vi "Scan Engine EtherCAT Slave.vi"(8 "error in (no error)":errorcluster, 11 "Node Ptr":T1 format="%.0x") -> (0 "error out":errorcluster)   [LabVIEW 2016, in "Scan Engine Custom Device.lvlib"]
uses:
  Scan Engine Custom Device.lvlib
  <vilib>/NI Veristand/Custom Device API/Custom Device Item Ref.ctl
  <vilib>/NI Veristand/Custom Device API/Custom Device API.lvlib
panel:
  in  "Prepend":bool caption="Prepend slave position to name"
  in  "SHDocVw.IWebBrowser2":refnum<k7>(container)
  in  "Slave Position":u16
  in  "Header":cluster{"Section Name":string}={"Section Name"="NI-9144 Chassis"}
  in  "Name":string
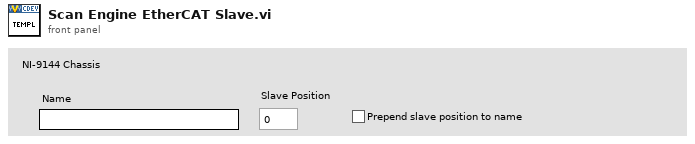
[diagram p1: front panel]
types:
  T1 = typedef "Custom Device API.lvlib/Custom Device Item Ref.ctl" = u64
  T2 = typedef "Custom Device API.lvlib/Custom Device Commands.ctl" = enum16{"Default", "Item renamed", "Shutdown", "Dynamic button pressed"}
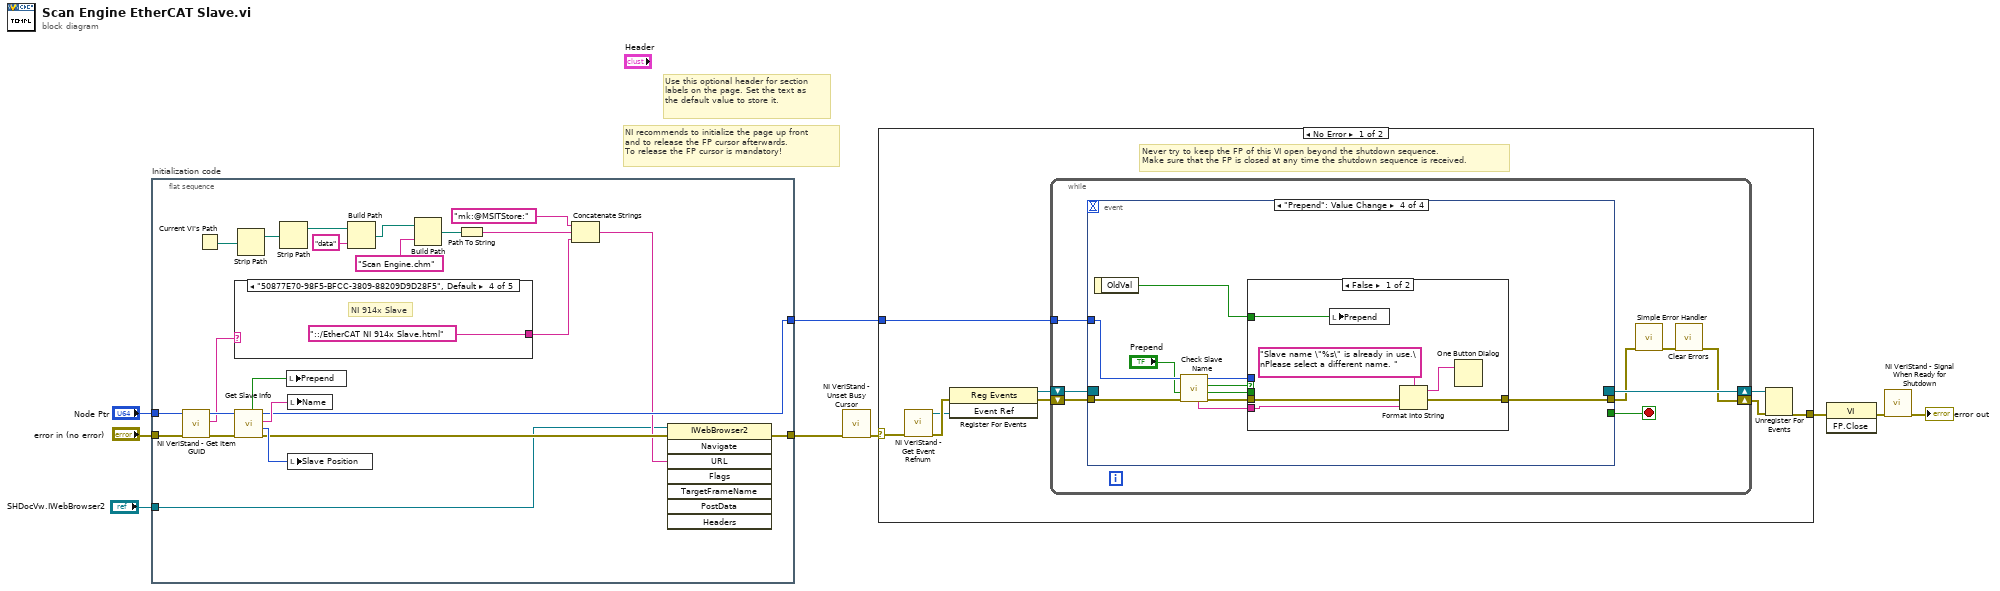
[diagram p0: block diagram]
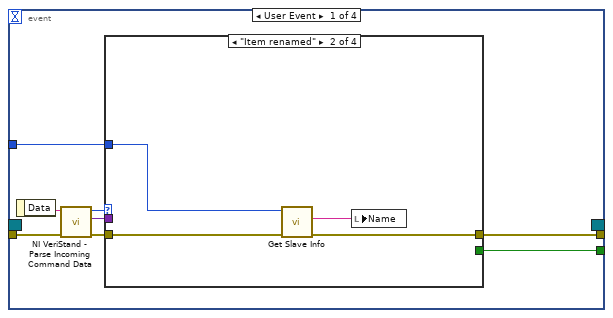
[diagram p2: hidden frame]
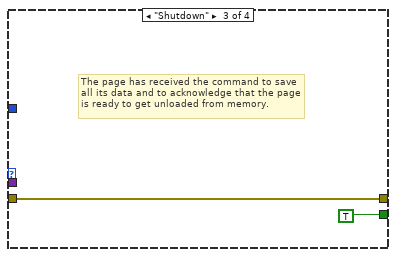
[diagram p4: hidden frame]
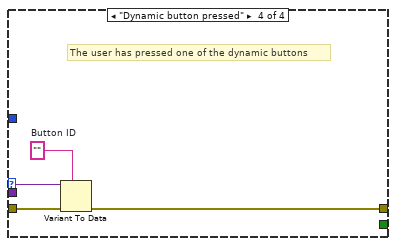
[diagram p5: hidden frame]
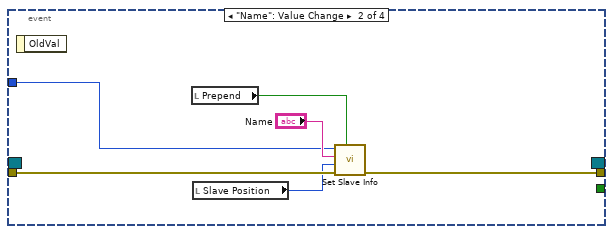
[diagram p6: hidden frame]
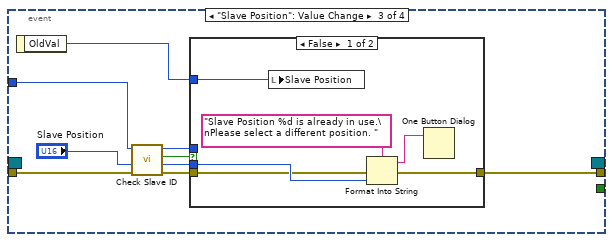
[diagram p7: hidden frame]
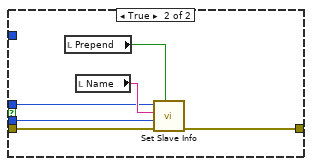
[diagram p8: hidden frame]
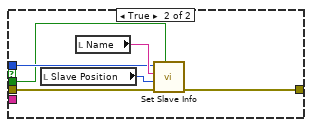
[diagram p9: hidden frame]
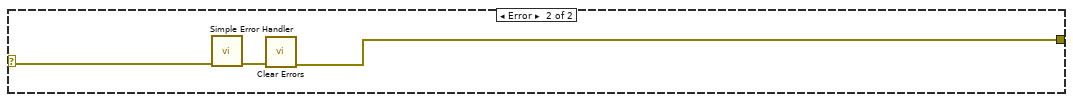
[diagram p10: hidden frame]
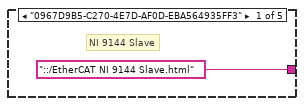
[diagram p11: hidden frame]
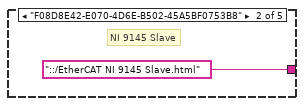
[diagram p12: hidden frame]
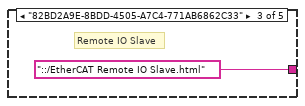
[diagram p13: hidden frame]
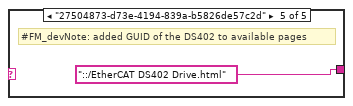
[diagram p14: hidden frame]
diagram:
  # "Use this optional header for section labels on the page. Set the text as the default value to store it."
  # "NI recommends to initialize the page up front\nand to release the FP cursor afterwards.\nTo release the FP cursor is mandatory!"
  n1 = flat-sequence "Initialization code" {
    tunnel: "error in (no error)" -> [w29]
    tunnel: "Node Ptr" -> [w13]
    tunnel: [w18] -> w5
    tunnel: [w30] -> w2
    tunnel: "SHDocVw.IWebBrowser2" -> [w16]
    frame #0 {
      n2 = call <vilib>:"NI VeriStand - Get Item GUID.vi"("error in (no error)"=w29, "Item Ref in"=w13) -> ("error out"=w14:errorcluster, "GUID"=w11:string, "Item Ref out"=w12:T1)  [unwired: 7 in]
      n3 = Current VI's Path() -> (path=w20:path)
      n4 = case shown="\"50877E70-98F5-BFCC-3809-88209D9D28F5\", Default" w11 {
        tunnel: ["::/EtherCAT NI 9144 Slave.html" ("name or relative path") "::/EtherCAT NI 9145 Slave.html" ("name or relative path") "::/EtherCAT Remote IO Slave.html" ("name or relative path") "::/EtherCAT NI 914x Slave.html" ("name or relative path") "::/EtherCAT DS402 Drive.html" ("name or relative path")] -> w10
        frame "0967D9B5-C270-4E7D-AF0D-EBA564935FF3" {
          # "NI 9144 Slave"
        }
        frame "F08D8E42-E070-4D6E-B502-45A5BF0753B8" {
          # "NI 9145 Slave"
        }
        frame "82BD2A9E-8BDD-4505-A7C4-771AB6862C33" {
          # "Remote IO Slave"
        }
        frame "50877E70-98F5-BFCC-3809-88209D9D28F5", Default {
          # "NI 914x Slave"
        }
        frame "27504873-d73e-4194-839a-b5826de57c2d" {
          # "#FM_devNote: added GUID of the DS402 to available pages"
        }
      }
      n5 = call "Get Slave Info.vi"("error in (no error)"=w14, "Item Ref in"=w12) -> ("error out"=w19:errorcluster, "Slave #"=w31:u16, "Slave Name"=w32:string, "Item Ref out"=w30:T1, "Prepend"=w15:bool)  [unwired: 5 in]
      n6 = Strip Path(path=w20) -> (stripped path=w21:path)  [unwired: 1 out]
      n7 = Strip Path(path=w21) -> (stripped path=w26:path)  [unwired: 1 out]
      n8 = local write "Prepend"(w15) -> ()
      n9 = local write "Name"(w32) -> ()
      n10 = local write "Slave Position"(w31) -> ()
      n11 = Build Path(base path=w26, name or relative path="data") -> (appended path=w27:path)
      n12 = Build Path(base path=w27, name or relative path="Scan Engine.chm") -> (appended path=w24:path)
      n13 = Path To String(path=w24) -> (string=w23:string)
      n14 = Concatenate Strings("mk:@MSITStore:" ("string"), w23, w10) -> (w17:string)
      n15 = invoke class="IWebBrowser2" method="Navigate"(reference=w16, error in=w19, "URL"=w17) -> (error out=w18:errorcluster)  [unwired: 5 in, 7 out]
    }
  }
  n16 = call <vilib>:"NI VeriStand - Unset Busy Cursor.vi"("error in (no error)"=w5) -> ("error out"=w4:errorcluster)  [unwired: 10 out]
  n17 = case shown="No Error" w4 {
    selector: w4 -> [w38 w125]
    tunnel: [w43 w123] -> w9
    tunnel: w2 -> [w39 _]
    frame No Error {
      # "Never try to keep the FP of this VI open beyond the shutdown sequence.\nMake sure that the FP is closed at any time the shutdown sequence is received."
      n18 = call <vilib>:"NI VeriStand - Get Event Refnum.vi"("error in (no error)"=w38) -> ("error out"=w46:errorcluster, "Event Ref"=w42:refnum<user-event>)  [unwired: 9 out]
      n19 = register-events(error in=w46, w42) -> (reference out=w40:refnum<event-registration>, error out=w41:errorcluster)  [unwired: 1 in]
      n20 = while {
        tunnel: w39 -> [w50]
        shift-right: [w47] -> w44
        shift-left: w41 -> [w53]
        shift-right: [w54] -> w45
        shift-left: w40 -> [w52]
        stop <- w51 stop-if-true
        n21 = event shown="[3] \"Prepend\": Value Change" {
          selector: w52 -> [_ _ _ _]
          dyn-events: [_ _ _ _] -> w54
          timeout: _ -> [_ _ _ _]
          tunnel: w53 -> [w62 w77 w82 w108]
          tunnel: [w58 _ _ _] -> w51
          tunnel: [w57 w78 w80 w109] -> w49
          tunnel: w50 -> [w56 w76 w84 w107]
          event User Event {
            n22 = event-data() -> ("Data"=w61:string)  [unwired: 1 out]
            n23 = call <vilib>:"NI VeriStand - Parse Incoming Command Data.vi"("error in (no error)"=w62, "Incoming data"=w61) -> ("error out"=w60:errorcluster, "Outgoing data"=w55:variant, "Action"=w59:T2)  [unwired: 7 out]
            n24 = case shown="\"Item renamed\"" w59 {
              tunnel: w60 -> [w63 w67 w68 w73]
              tunnel: [_ _ TRUE _] -> w58
              tunnel: [w63 w66 w68 w70] -> w57
              tunnel: w56 -> [_ w64 _ _]
              tunnel: w55 -> [_ _ _ w72]
              frame "Default", Default {
              }
              frame "Item renamed" {
                n25 = call "Get Slave Info.vi"("error in (no error)"=w67, "Item Ref in"=w64) -> ("error out"=w66:errorcluster, "Slave Name"=w65:string)  [unwired: 5 in, 3 out]
                n26 = local write "Name"(w65) -> ()
              }
              frame "Shutdown" {
                # "The page has received the command to save all its data and to acknowledge that the page is ready to get unloaded from memory."
              }
              frame "Dynamic button pressed" {
                w71 = ""  # Button ID
                # "The user has pressed one of the dynamic buttons"
                n27 = Variant To Data(error in=w73, type=w71, Variant=w72) -> (error out=w70:errorcluster)  [unwired: 1 out]
              }
            }
          }
          event "Name": Value Change {
            n28 = event-data() -> ()  [unwired: 2 out]
            n29 = local read "Prepend"() -> (w74:bool)
            n30 = local read "Slave Position"() -> (w75:u16)
            n31 = call "Set Slave Info.vi"("Prepend"=w74, "error in (no error)"=w77, "Slave #"=w75, "Slave Name"="Name", "Item Ref in"=w76) -> ("error out"=w78:errorcluster)  [unwired: 5 in, 1 out]
          }
          event "Slave Position": Value Change {
            n32 = event-data() -> ("OldVal"=w81:u16)  [unwired: 1 out]
            n33 = call "Check Slave ID.vi"("error in (no error)"=w82, "Slave ID in"="Slave Position", "Item Ref in"=w84) -> ("error out"=w88:errorcluster, "Slave ID out"=w86:u16, "Available?"=w87:bool, "Item Ref out"=w85:T1)  [unwired: 5 in]
            n34 = case shown="False" w87 {
              tunnel: [w90 w100] -> w80
              tunnel: w88 -> [w91 w99]
              tunnel: w85 -> [_ w96]
              tunnel: w86 -> [w93 w98]
              tunnel: w81 -> [w89 _]
              frame False {
                n35 = local write "Slave Position"(w89) -> ()
                n36 = Format Into String(format string="Slave Position %d is already in use.\nPlease select a different position. ", error in=w91, w93) -> (resulting string=w92:string, error out=w90:errorcluster)  [unwired: 1 in]
                n37 = One Button Dialog(message=w92) -> ()  [unwired: 1 in, 1 out]
              }
              frame True {
                n38 = local read "Prepend"() -> (w95:bool)
                n39 = local read "Name"() -> (w97:string)
                n40 = call "Set Slave Info.vi"("Prepend"=w95, "error in (no error)"=w99, "Slave #"=w98, "Slave Name"=w97, "Item Ref in"=w96) -> ("error out"=w100:errorcluster)  [unwired: 5 in, 1 out]
              }
            }
          }
          event "Prepend": Value Change {
            n41 = event-data() -> ("OldVal"=w110:bool)  [unwired: 1 out]
            n42 = call "Check Slave Name.vi"("error in (no error)"=w108, "Prepend in"="Prepend", "Item Ref in"=w107) -> ("error out"=w103:errorcluster, "Prepend out"=w102:bool, "Available?"=w104:bool, "Item Ref out"=w105:T1, "Slave Name"=w101:string)  [unwired: 4 in]
            n43 = case shown="False" w104 {
              tunnel: [w113 w122] -> w109
              tunnel: w103 -> [w114 w121]
              tunnel: w105 -> [_ w119]
              tunnel: w102 -> [_ w118]
              tunnel: w110 -> [w116 _]
              tunnel: w101 -> [w111 _]
              frame False {
                n44 = local write "Prepend"(w116) -> ()
                n45 = Format Into String(format string="Slave name \"%s\" is already in use.\nPlease select a different name. ", error in=w114, w111) -> (resulting string=w112:string, error out=w113:errorcluster)  [unwired: 1 in]
                n46 = One Button Dialog(message=w112) -> ()  [unwired: 1 in, 1 out]
              }
              frame True {
                n47 = local read "Slave Position"() -> (w117:u16)
                n48 = local read "Name"() -> (w120:string)
                n49 = call "Set Slave Info.vi"("Prepend"=w118, "error in (no error)"=w121, "Slave #"=w117, "Slave Name"=w120, "Item Ref in"=w119) -> ("error out"=w122:errorcluster)  [unwired: 5 in, 1 out]
              }
            }
          }
        }
        n50 = call <vilib>:"Simple Error Handler.vi"("error in (no error)"=w49) -> ("error out"=w48:errorcluster)  [unwired: 1 in, 7 out]
        n51 = call <vilib>:"Clear Errors.vi"("error in (no error)"=w48) -> ("error out"=w47:errorcluster)  [unwired: 1 in, 5 out]
      }
      n52 = Unregister For Events(event registration refnum=w45, error in=w44) -> (error out=w43:errorcluster)
    }
    frame Error {
      n53 = call <vilib>:"Simple Error Handler.vi"("error in (no error)"=w125) -> ("error out"=w124:errorcluster)  [unwired: 1 in, 7 out]
      n54 = call <vilib>:"Clear Errors.vi"("error in (no error)"=w124) -> ("error out"=w123:errorcluster)  [unwired: 1 in, 5 out]
    }
  }
  n55 = invoke class="VI" method="FP.Close"(error in=w9) -> (error out=w8:errorcluster)  [unwired: 2 in, 2 out]
  n56 = call <vilib>:"NI VeriStand - Signal When Ready for Shutdown.vi"("error in (no error)"=w8) -> ("error out"=→"error out":errorcluster)  [unwired: 10 out]
